vi "Set Enable State Boolean.vi"(8 "error in (no error)":errorcluster, 9 "Enable State":T1(ring), 11 "Boolean Ref Array":refnum<vi>[](array[refnum])) -> (0 "error out":errorcluster, 3 "Boolean Ref Array":refnum<vi>[](array[refnum]))   [LabVIEW 2014]
doc: "<B>Copyright</B>: (c) MHWirth 2015. All rights are reserved.\n\nThis SubVI sets the control/indicators enable/disable. \nIt accepts an array of references (only for DBL type)."
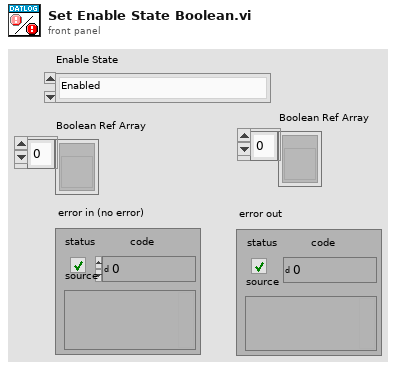
[diagram p1: front panel]
types:
  T1 = enum8{"Enabled", "Disabled", "Disabled and Grayed Out"}
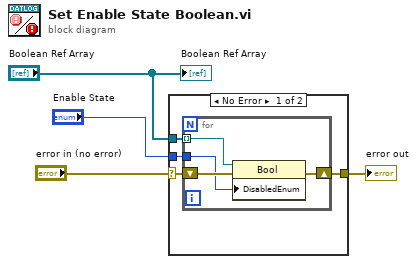
[diagram p0: block diagram]
diagram:
  n1 = case shown="No Error" "error in (no error)" {
    selector: "error in (no error)" -> [w8 w13]
    tunnel: [w7 w13] -> w3
    tunnel: "Enable State" -> [w6 _]
    tunnel: "Boolean Ref Array" -> [w5 _]
    frame No Error {
      n2 = for {
        shift-right: [w11] -> w7
        shift-left: w8 -> [w12]
        tunnel: w6 -> [w10]
        tunnel: w5 -> [w9] mode=indexing
        n3 = property class="Bool"(reference=w9, error in=w12, "DisabledEnum"=w10) -> (error out=w11:errorcluster)  [unwired: 1 out]
      }
    }
    frame Error {
    }
  }
  "error out" <- w3
  "Boolean Ref Array" <- "Boolean Ref Array"
